vi "DataInit.vi"() -> (3 "output cluster":T1)   [LabVIEW 2011]
uses:
  MainCluster_typdef.ctl
  EC Status Named_typdef.ctl
  EC Statusboolarray2_typdef.ctl
  EC Statusboolarray3_typdef.ctl
  EC Statusboolarray1_typdef.ctl
  EC statusintegerarray_typdef.ctl
  EC statusfloatrarray_typdef.ctl
  LB Status Named_typdef.ctl
  LB Statusboolarray1_typdef.ctl
  LB Statusboolarray2_typdef.ctl
  LB Statusboolarray3_typdef.ctl
  LB statusintegerarray_typdef.ctl
  LB statusfloatrarray_typdef.ctl
  Chamber Selection_typdef.ctl
  GPM Mode_typdef.ctl
panel:
  in  "LB Status Named":T16
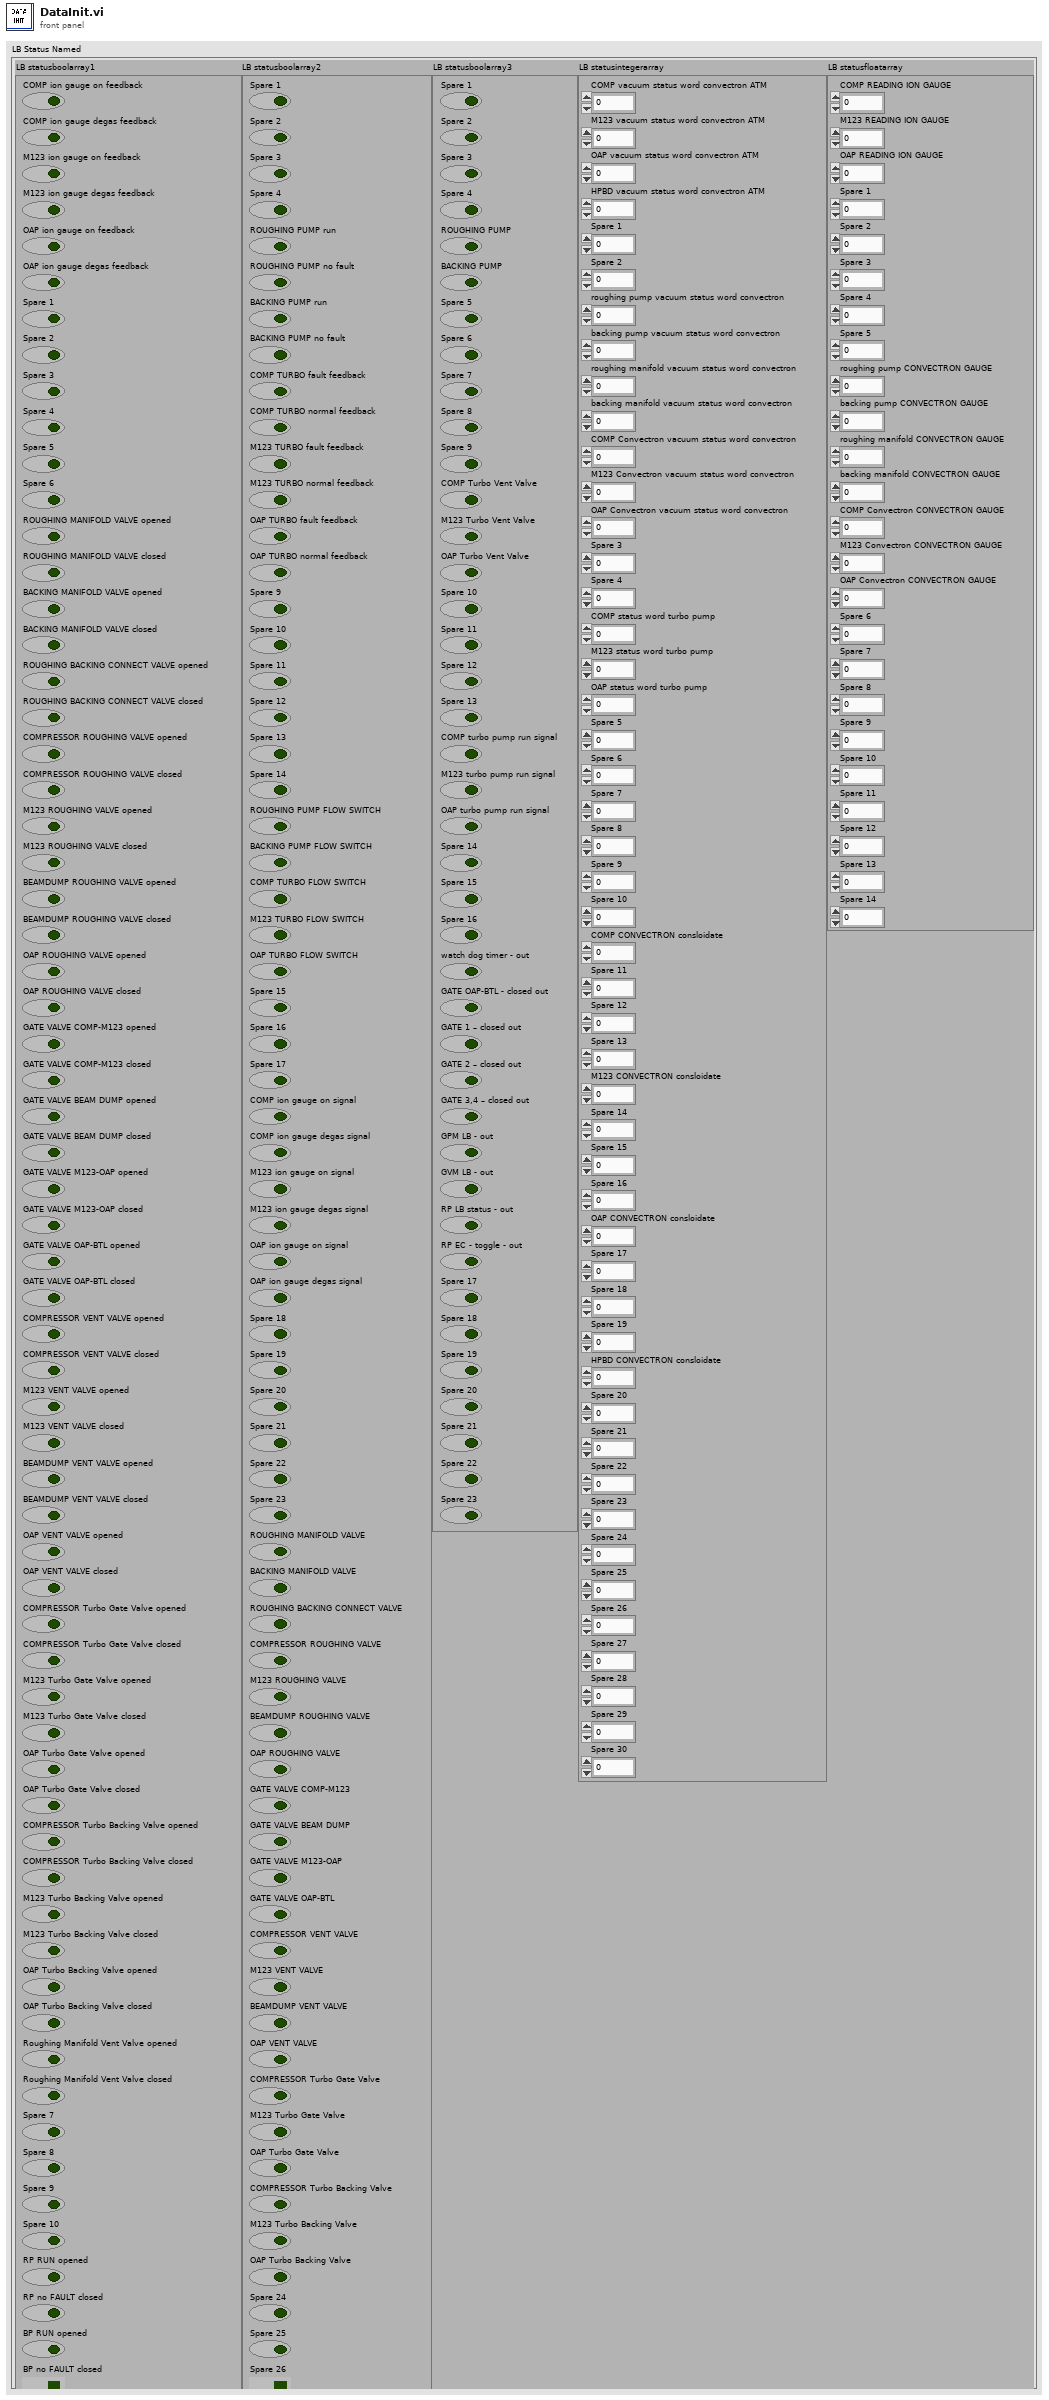
[diagram p1: front panel]
types:
  T1 = typedef "MainCluster_typdef.ctl" = cluster{"Isolate HPBD":bool, "Core":cluster{"Current VI Reference":refnum<vi>, "Close Panel on Exit?":bool}, "Status Display Array":string[], "Connection URLs":cluster{"Source_URL EC":string, "Target_URL EC":string, "Source_URL LB":string, "Target_URL LB":string}, "EC Status":cluster{"bits 2":bool[], "bits 2":bool[], "bits 2":bool[], i32[], "FLOAT NUMBERS 2":sgl[]}, "EC Status Named":T2, "TCPConnection":cluster{"Status TCP Connection EC":refnum<k5>, "Command TCP Connection EC":refnum<k5>, "Status TCP Connection LB":refnum<k5>, "Command TCP Connection LB":refnum<k5>}, "EC Command Cluster":cluster{"boolarray1":cluster{bool, bool, bool, bool, bool, bool, bool, bool, bool, bool, bool, bool, bool, bool, bool, bool}, "boolarray2":cluster{bool, bool, bool, bool, bool, bool, bool, bool, bool, bool, bool, bool, bool, bool, bool, bool}, "boolarray3":cluster{bool, bool, bool, bool, bool, bool, bool, bool, bool, bool, bool, bool, bool, bool, bool, bool}, "boolarray4":cluster{bool, bool, bool, bool, bool, bool, bool, bool, bool, bool, bool, bool, bool, bool, bool, bool}}, "EC Command Named":cluster{"EC Command array 1":cluster{"ROUGHING MANIFOLD VALVE":bool, "BACKING MANIFOLD VALVE":bool, "ROUGHING BACKING CONNECT VALVE":bool, "BTL ROUGHING VALVE":bool, "BTL VENT VALVE":bool, "BTL Turbo Gate Valve":bool, "BTL Turbo Backing Valve":bool, "Roughing Manifold VV":bool, "Backing Manifold VV":bool, "TARGET ROUGHING VALVE":bool, "BTL2 ROUGHING VALVE":bool, "HPD ROUGHING VALVE":bool, "GV BTL-TARGET":bool, "GV TARGET-BTL2":bool, "GV BTL2-HPD":bool, "TARGET VENT VALVE":bool}, " EC Command array 2":cluster{"BTL2 VENT VALVE":bool, "HPD VENT VALVE":bool, "TARGET  Turbo Gate Valve 1":bool, "TARGET  Turbo Gate Valve 2":bool, "BTL2 Turbo Gate Valve":bool, "HPD  Turbo Gate Valve":bool, "TARGET Turbo Backing Valve 1":bool, "TARGET Turbo Backing Valve 2":bool, "BTL2 Turbo Backing Valve":bool, "HPD Turbo Backing Valve":bool, "Spare 1":bool, "Spare 2":bool, "ROUGHING PUMP":bool, "BACKING PUMP":bool, "Spare 3":bool, "Spare 4":bool}, "EC Command array 3":cluster{"Spare 1":bool, "Spare 2":bool, "Spare 3":bool, "BTL Turbo Vent Valve":bool, "TARGET1 Turbo Vent Valve":bool, "TARGET2 Turbo Vent Valve":bool, "BTL2 Turbo Vent Valve":bool, "HPD Turbo Vent Valve":bool, "Spare 4":bool, "Spare 5":bool, "GPM":bool, "GVM":bool, "Spare 6":bool, "BTL turbo pump":bool, "TARGET1 turbo pump":bool, "TARGET2 turbo pump":bool}, "EC Command array 4":cluster{"BLT turbo pump":bool, "HPD turbo pump":bool, "Spare 1":bool, "BTL ION GAUGE ion gauge":bool, "BTL ION GAUGE  ion gauge degas":bool, "TARGET ion gauge":bool, "TARGET ion gauge degas":bool, "BTL2 ion gauge":bool, "BTL2 ion gauge degas":bool, "HPD ion gauge":bool, "HPD ion gauge degas":bool, "Spare 2":bool, "Spare 3":bool, "Spare 4":bool, "Spare 5":bool, "Spare 6":bool}}, "LB Status Named":T8, "LB Status":cluster{"bits 2":bool[], "bits 2":bool[], "bits 2":bool[], i32[], "FLOAT NUMBERS 2":sgl[]}, "LB Command Cluster":cluster{"boolarray1":cluster{bool, bool, bool, bool, bool, bool, bool, bool, bool, bool, bool, bool, bool, bool, bool, bool}, "boolarray2":cluster{bool, bool, bool, bool, bool, bool, bool, bool, bool, bool, bool, bool, bool, bool, bool, bool}, "boolarray3":cluster{bool, bool, bool, bool, bool, bool, bool, bool, bool, bool, bool, bool, bool, bool, bool, bool}, "boolarray4":cluster{bool, bool, bool, bool, bool, bool, bool, bool, bool, bool, bool, bool, bool, bool, bool, bool}}, "LB Command Named":cluster{"LB commandarray1":cluster{"ROUGHING MANIFOLD VALVE":bool, "BACKING MANIFOLD VALVE":bool, "ROUGHING BACKING CONNECT VALVE":bool, "COMPRESSOR ROUGHING VALVE":bool, "M123 ROUGHING VALVE":bool, "BEAMDUMP ROUGHING VALVE":bool, "OAP ROUGHING VALVE":bool, "GATE VALVE COMP-M123":bool, "GATE VALVE BEAM DUMP":bool, "GATE VALVE M123-OAP":bool, "GATE VALVE OAP-BTL":bool, "COMPRESSOR VENT VALVE":bool, "M123 VENT VALVE":bool, "BEAMDUMP VENT VALVE":bool, "OAP VENT VALVE":bool, "COMPRESSOR Turbo Gate Valve":bool}, "LB commandarray2":cluster{"M123 Turbo Gate Valve":bool, "OAP Turbo Gate Valve":bool, "COMPRESSOR Turbo Backing Valve":bool, "M123 Turbo Backing Valve":bool, "OAP Turbo Backing Valve":bool, "Roughing Manifold Vent Valve":bool, "Backing Manifold Vent Valve":bool, "Spare 1":bool, "Spare 2":bool, "Spare 3":bool, "Spare 4":bool, "Spare 5":bool, "ROUGHING PUMP":bool, "BACKING PUMP":bool, "Spare 6":bool, "Spare 7":bool}, "LB commandarray3":cluster{"Spare 1":bool, "Spare 2":bool, "Spare 3":bool, "COMP Turbo Vent Valve":bool, "M123 Turbo Vent Valve":bool, "OAP Turbo Vent Valve":bool, "Spare 4":bool, "Spare 5":bool, "Spare 6":bool, "Spare 7":bool, "GPM":bool, "GVM":bool, "Spare 8":bool, "COMP turbo pump":bool, "M123 turbo pump":bool, "OAP turbo pump":bool}, "LB commandarray4":cluster{"Spare 1":bool, "Spare 2":bool, "Spare 3":bool, "COMP ION GAUGE":bool, "COMP ION GAUGE degas":bool, "M123 ION GAUGE":bool, "M123 ION GAUGE degas":bool, "OAP ION GAUGE":bool, "OAP ION GAUGE degas":bool, "Spare 4":bool, "Spare 5":bool, "Spare 6":bool, "Spare 7":bool, "Spare 8":bool, "Spare 9":bool, "Spare 10":bool}}, "VI Refnum":refnum<vi>, "Chamber Selection":T14, "GPM Mode":T15, "Debug Mode?":bool, "State Sanity Check Array":bool[], "Critical Failures":cluster{"GPM Exit?":bool}, "Comm Ready?":bool, "Status Reconnect Attempt":dbl}
  T2 = typedef "EC Status Named_typdef.ctl" = cluster{"EC statusboolarray2":T3, "EC statusboolarray3":T4, "EC statusboolarray1":T5, "EC statusintegerarray":T6, "EC statusfloatarray":T7}
  T3 = typedef "EC Statusboolarray2_typdef.ctl" = cluster{"Spare 1":bool, "Spare 2":bool, "Spare 3":bool, "Spare 4":bool, "ROUGHING PUMP run opened":bool, "ROUGHING PUMP no fault closed":bool, "BACKING PUMP run opened":bool, "BACKING PUMP no fault closed":bool, "BTL TURBO turbo fault feedback":bool, "BTL TURBO turbo normal feedback":bool, "TARGET 1 TURBO turbo fault feedback":bool, "TARGET 1 TURBO turbo normal feedback":bool, "TARGET 2 TURBO turbo fault feedback":bool, "TARGET 2 TURBO turbo normal feedback":bool, "BTL2 TURBO turbo fault feedback":bool, "BTL2 TURBO turbo normal feedback":bool, "HPD TURBO turbo fault feedback":bool, "HPD TURBO turbo normal feedback":bool, "Spare 5":bool, "Spare 6":bool, "ROUGHING PUMP FLOW SWITCH":bool, "BACKING PUMP FLOW SWITCH":bool, "BTL TURBO FLOW SWITCH":bool, "TARGET 1 TURBO FLOW SWITCH":bool, "TARGET 2 TURBO FLOW SWITCH":bool, "BTL2 TURBO FLOW SWITCH":bool, "HPD TURBO FLOW SWITCH":bool, "Spare 7":bool, "BTL ion gauge on signal":bool, "BTL ion gauge degas signal":bool, "TARGET ion gauge on signal":bool, "TARGET ion gauge degas signal":bool, "BTL2 ion gauge on signal":bool, "BTL2 ion gauge degas signal":bool, "HPD ion gauge on signal":bool, "HPD ion gauge degas signal":bool, "Spare 8":bool, "Spare 9":bool, "Spare 10":bool, "Spare 11":bool, "ROUGHING MANIFOLD VALVE":bool, "BACKING MANIFOLD VALVE":bool, "ROUGHING BACKING CONNECT VALVE":bool, "BTL ROUGHING VALVE":bool, "BTL VENT VALVE":bool, "BTL Turbo Gate Valve":bool, "BTL Turbo Backing Valve":bool, "Roughing Manifold VV":bool, "Backing Manifold VV":bool, "TARGET ROUGHING VALVE":bool, "BTL2 ROUGHING VALVE":bool, "HPD ROUGHING VALVE":bool, "GV BTL-TARGET":bool, "GV TARGET-BTL2":bool, "GV BTL2-HPD":bool, "TARGET VENT VALVE":bool, "BTL2 VENT VALVE":bool, "HPD VENT VALVE":bool, "TARGET  Turbo Gate Valve 1":bool, "TARGET  Turbo Gate Valve 2":bool, "BTL2 Turbo Gate Valve":bool, "HPD  Turbo Gate Valve":bool, "TARGET Turbo Backing Valve 1":bool, "TARGET Turbo Backing Valve 2":bool}
  T4 = typedef "EC Statusboolarray3_typdef.ctl" = cluster{"BTL2 Turbo Backing Valve":bool, "HPD Turbo Backing Valve":bool, "Spare 1":bool, "Spare 2":bool, "Spare 3":bool, "Spare 4":bool, "Spare 5":bool, "Spare 6":bool, "Spare 7":bool, "Spare 8":bool, "Spare 9":bool, "BTL Turbo Vent Valve":bool, "TARGET1 Turbo Vent Valve":bool, "TARGET2 Turbo Vent Valve":bool, "BTL2 Turbo Vent Valve":bool, "HPD Turbo Vent Valve":bool, "Spare 10":bool, "Spare 11":bool, "BTL turbo pump run signal":bool, "TARGET1 turbo pump run signal":bool, "TARGET2 turbo pump run signal":bool, "BTL2 turbo pump run signal":bool, "HPD turbo pump run signal":bool, "Spare 12":bool, "watch dog timer - out":bool, "BTL vented – out":bool, "BTL medvac – out":bool, "BTL hivac – out":bool, "GPM EC - out":bool, "GVM EC - out":bool, "RP EC status - out":bool, "RP LB toggle - out":bool, "GATE ALL - closed out":bool, "Spare 13":bool, "Spare 14":bool, "Spare 15":bool, "Spare 16":bool, "Spare 17":bool, "Spare 18":bool, "Spare 19":bool, "Spare 20":bool, "Spare 21":bool, "Spare 22":bool, "Spare 23":bool, "Spare 24":bool, "Spare 25":bool, "Spare 26":bool, "Spare 27":bool}
  T5 = typedef "EC Statusboolarray1_typdef.ctl" = cluster{"BTL ion gauge on feedback":bool, "BTL ion gauge degas feedback":bool, "TARGET ion gauge on feedback":bool, "TARGET ion gauge degas feedback":bool, "BTL2 ion gauge on feedback":bool, "BTL2 ion gauge degas feedback":bool, "HPD ion gauge on feedback":bool, "HPD ion gauge degas feedback":bool, "Spare 1":bool, "Spare 2":bool, "Spare 3":bool, "Spare 4":bool, "ROUGHING MANIFOLD VALVE opened":bool, "ROUGHING MANIFOLD VALVE closed":bool, "BACKING MANIFOLD VALVE opened":bool, "BACKING MANIFOLD VALVE closed":bool, "ROUGHING BACKING CONNECT VALVE opened":bool, "ROUGHING BACKING CONNECT VALVE closed":bool, "BTL ROUGHING VALVE opened":bool, "BTL ROUGHING VALVE closed":bool, "BTL VENT VALVE opened":bool, "BTL VENT VALVE closed":bool, "BTL Turbo Gate Valve opened":bool, "BTL Turbo Gate Valve closed":bool, "BTL Turbo Backing Valve opened":bool, "BTL Turbo Backing Valve closed":bool, "Roughing Manifold VV opened":bool, "Roughing Manifold VV closed":bool, "Backing Manifold VV opened":bool, "Backing Manifold VV closed":bool, "TARGET ROUGHING VALVE opened":bool, "TARGET ROUGHING VALVE closed":bool, "BTL2 ROUGHING VALVE opened":bool, "BTL2 ROUGHING VALVE closed":bool, "HPD ROUGHING VALVE opened":bool, "HPD ROUGHING VALVE closed":bool, "GV BTL-TARGET opened":bool, "GV BTL-TARGET closed":bool, "GV TARGET-BTL2 opened":bool, "GV TARGET-BTL2 closed":bool, "GV BTL2-HPD opened":bool, "GV BTL2-HPD closed":bool, "TARGET VENT VALVE opened":bool, "TARGET VENT VALVE closed":bool, "BTL2 VENT VALVE opened":bool, "BTL2 VENT VALVE closed":bool, "HPD VENT VALVE opened":bool, "HPD VENT VALVE closed":bool, "TARGET  Turbo Gate Valve 1 opened":bool, "TARGET  Turbo Gate Valve 1 closed":bool, "TARGET  Turbo Gate Valve 2 opened":bool, "TARGET  Turbo Gate Valve 2 closed":bool, "BTL2 Turbo Gate Valve opened":bool, "BTL2 Turbo Gate Valve closed":bool, "HPD  Turbo Gate Valve opened":bool, "HPD  Turbo Gate Valve closed":bool, "TARGET Turbo Backing Valve 1 opened":bool, "TARGET Turbo Backing Valve 1 closed":bool, "TARGET Turbo Backing Valve 2 opened":bool, "TARGET Turbo Backing Valve 2 closed":bool, "BTL2 Turbo Backing Valve opened":bool, "BTL2 Turbo Backing Valve closed":bool, "HPD Turbo Backing Valve opened":bool, "HPD Turbo Backing Valve closed":bool}
  T6 = typedef "EC statusintegerarray_typdef.ctl" = cluster{"BTL vacuum status word convectron ATM":i32, "TARGET vacuum status word convectron ATM 2":i32, "BTL2 vacuum status word convectron ATM 3":i32, "HPD vacuum status word convectron ATM 4":i32, "Spare 1":i32, "Spare 2":i32, "roughing pump vacuum status word convectron":i32, "backing pump vacuum status word convectron":i32, "roughing manifold vacuum status word convectron":i32, "backing manifold vacuum status word convectron":i32, "BTL Convectron vacuum status word convectron":i32, "TARGET1 Convectron vacuum status word convectron":i32, "TARGET2 Convectron vacuum status word convectron":i32, "BTL2 Convectron vacuum status word convectron":i32, "HPD Convectron vacuum status word convectron":i32, "BTL status word turbo pump":i32, "TARGET1 status word turbo pump":i32, "TARGET2 status word turbo pump":i32, "BTL2 status word turbo pump??":i32, "HPD status word turbo pump":i32, "Spare 3":i32, "Spare 4":i32, "Spare 5":i32, "Spare 6":i32, "BTL CONVECTRON Consolidate":i32, "Spare 7":i32, "Spare 8":i32, "Spare 9":i32, "TARGET Consolidate":i32, "Spare 10":i32, "Spare 11":i32, "Spare 12":i32, "BTL2 Consolidate":i32, "Spare 13":i32, "Spare 14":i32, "Spare 15":i32, "HPD Consolidate":i32, "Spare 16":i32, "Spare 17":i32, "Spare 18":i32, "Spare 19":i32, "Spare 20":i32, "Spare 21":i32, "Spare 22":i32, "Spare 23":i32, "Spare 24":i32, "Spare 25":i32, "Spare 26":i32}
  T7 = typedef "EC statusfloatrarray_typdef.ctl" = cluster{"BTL READING ION GAUGE":dbl, "TARGET READING ION GAUGE":dbl, "BTL2 READING ION GAUGE":dbl, "HPD READING ION GAUGE":dbl, "Spare 1":dbl, "Spare 2":dbl, "Spare 3":dbl, "Spare 4":dbl, "roughing pump READING CONVECTRON GAUGE":dbl, "backing pump READING CONVECTRON GAUGE":dbl, "roughing manifold READING CONVECTRON GAUGE":dbl, "backing manifold READING CONVECTRON GAUGE":dbl, "BTL Convectron READING CONVECTRON GAUGE":dbl, "TARGET1 READING CONVECTRON GAUGE":dbl, "TARGET2 READING CONVECTRON GAUGE":dbl, "BTL2 READING CONVECTRON GAUGE":dbl, "HPD READING CONVECTRON GAUGE":dbl, "Spare 5":dbl, "Spare 6":dbl, "Spare 7":dbl, "Spare 8":dbl, "Spare 9":dbl, "Spare 10":dbl, "Spare 11":dbl}
  T8 = typedef "LB Status Named_typdef.ctl" = cluster{"LB statusboolarray1":T9, "LB statusboolarray2":T10, "LB statusboolarray3":T11, "LB statusintegerarray":T12, "LB statusfloatarray":T13}
  T9 = typedef "LB Statusboolarray1_typdef.ctl" = cluster{"COMP ion gauge on feedback":bool, "COMP ion gauge degas feedback":bool, "M123 ion gauge on feedback":bool, "M123 ion gauge degas feedback":bool, "OAP ion gauge on feedback":bool, "OAP ion gauge degas feedback":bool, "Spare 1":bool, "Spare 2":bool, "Spare 3":bool, "Spare 4":bool, "Spare 5":bool, "Spare 6":bool, "ROUGHING MANIFOLD VALVE opened":bool, "ROUGHING MANIFOLD VALVE closed":bool, "BACKING MANIFOLD VALVE opened":bool, "BACKING MANIFOLD VALVE closed":bool, "ROUGHING BACKING CONNECT VALVE opened":bool, "ROUGHING BACKING CONNECT VALVE closed":bool, "COMPRESSOR ROUGHING VALVE opened":bool, "COMPRESSOR ROUGHING VALVE closed":bool, "M123 ROUGHING VALVE opened":bool, "M123 ROUGHING VALVE closed":bool, "BEAMDUMP ROUGHING VALVE opened":bool, "BEAMDUMP ROUGHING VALVE closed":bool, "OAP ROUGHING VALVE opened":bool, "OAP ROUGHING VALVE closed":bool, "GATE VALVE COMP-M123 opened":bool, "GATE VALVE COMP-M123 closed":bool, "GATE VALVE BEAM DUMP opened":bool, "GATE VALVE BEAM DUMP closed":bool, "GATE VALVE M123-OAP opened":bool, "GATE VALVE M123-OAP closed":bool, "GATE VALVE OAP-BTL opened":bool, "GATE VALVE OAP-BTL closed":bool, "COMPRESSOR VENT VALVE opened":bool, "COMPRESSOR VENT VALVE closed":bool, "M123 VENT VALVE opened":bool, "M123 VENT VALVE closed":bool, "BEAMDUMP VENT VALVE opened":bool, "BEAMDUMP VENT VALVE closed":bool, "OAP VENT VALVE opened":bool, "OAP VENT VALVE closed":bool, "COMPRESSOR Turbo Gate Valve opened ":bool, "COMPRESSOR Turbo Gate Valve closed":bool, "M123 Turbo Gate Valve opened":bool, "M123 Turbo Gate Valve closed":bool, "OAP Turbo Gate Valve opened":bool, "OAP Turbo Gate Valve closed":bool, "COMPRESSOR Turbo Backing Valve opened":bool, "COMPRESSOR Turbo Backing Valve closed":bool, "M123 Turbo Backing Valve opened":bool, "M123 Turbo Backing Valve closed":bool, "OAP Turbo Backing Valve opened":bool, "OAP Turbo Backing Valve closed":bool, "Roughing Manifold Vent Valve opened":bool, "Roughing Manifold Vent Valve closed":bool, "Spare 7":bool, "Spare 8":bool, "Spare 9":bool, "Spare 10":bool, "RP RUN opened":bool, "RP no FAULT closed":bool, "BP RUN opened":bool, "BP no FAULT closed":bool}
  T10 = typedef "LB Statusboolarray2_typdef.ctl" = cluster{"Spare 1":bool, "Spare 2":bool, "Spare 3":bool, "Spare 4":bool, "ROUGHING PUMP run":bool, "ROUGHING PUMP no fault":bool, "BACKING PUMP run":bool, "BACKING PUMP no fault":bool, "COMP TURBO fault feedback":bool, "COMP TURBO normal feedback":bool, "M123 TURBO fault feedback":bool, "M123 TURBO normal feedback":bool, "OAP TURBO fault feedback":bool, "OAP TURBO normal feedback":bool, "Spare 9":bool, "Spare 10":bool, "Spare 11":bool, "Spare 12":bool, "Spare 13":bool, "Spare 14":bool, "ROUGHING PUMP FLOW SWITCH":bool, "BACKING PUMP FLOW SWITCH":bool, "COMP TURBO FLOW SWITCH":bool, "M123 TURBO FLOW SWITCH":bool, "OAP TURBO FLOW SWITCH":bool, "Spare 15":bool, "Spare 16":bool, "Spare 17":bool, "COMP ion gauge on signal":bool, "COMP ion gauge degas signal":bool, "M123 ion gauge on signal":bool, "M123 ion gauge degas signal":bool, "OAP ion gauge on signal":bool, "OAP ion gauge degas signal":bool, "Spare 18":bool, "Spare 19":bool, "Spare 20":bool, "Spare 21":bool, "Spare 22":bool, "Spare 23":bool, "ROUGHING MANIFOLD VALVE":bool, "BACKING MANIFOLD VALVE":bool, "ROUGHING BACKING CONNECT VALVE":bool, "COMPRESSOR ROUGHING VALVE":bool, "M123 ROUGHING VALVE":bool, "BEAMDUMP ROUGHING VALVE":bool, "OAP ROUGHING VALVE":bool, "GATE VALVE COMP-M123":bool, "GATE VALVE BEAM DUMP":bool, "GATE VALVE M123-OAP":bool, "GATE VALVE OAP-BTL":bool, "COMPRESSOR VENT VALVE":bool, "M123 VENT VALVE":bool, "BEAMDUMP VENT VALVE":bool, "OAP VENT VALVE":bool, "COMPRESSOR Turbo Gate Valve":bool, "M123 Turbo Gate Valve":bool, "OAP Turbo Gate Valve":bool, "COMPRESSOR Turbo Backing Valve":bool, "M123 Turbo Backing Valve":bool, "OAP Turbo Backing Valve":bool, "Spare 24":bool, "Spare 25":bool, "Spare 26":bool}
  T11 = typedef "LB Statusboolarray3_typdef.ctl" = cluster{"Spare 1":bool, "Spare 2":bool, "Spare 3":bool, "Spare 4":bool, "ROUGHING PUMP":bool, "BACKING PUMP":bool, "Spare 5":bool, "Spare 6":bool, "Spare 7":bool, "Spare 8":bool, "Spare 9":bool, "COMP Turbo Vent Valve":bool, "M123 Turbo Vent Valve":bool, "OAP Turbo Vent Valve":bool, "Spare 10":bool, "Spare 11":bool, "Spare 12":bool, "Spare 13":bool, "COMP turbo pump run signal":bool, "M123 turbo pump run signal":bool, "OAP turbo pump run signal":bool, "Spare 14":bool, "Spare 15":bool, "Spare 16":bool, "watch dog timer - out":bool, "GATE OAP-BTL - closed out":bool, "GATE 1 – closed out":bool, "GATE 2 – closed out":bool, "GATE 3,4 – closed out":bool, "GPM LB - out":bool, "GVM LB - out":bool, "RP LB status - out":bool, "RP EC - toggle - out":bool, "Spare 17":bool, "Spare 18":bool, "Spare 19":bool, "Spare 20":bool, "Spare 21":bool, "Spare 22":bool, "Spare 23":bool}
  T12 = typedef "LB statusintegerarray_typdef.ctl" = cluster{"COMP vacuum status word convectron ATM":i32, "M123 vacuum status word convectron ATM":i32, "OAP vacuum status word convectron ATM":i32, "HPBD vacuum status word convectron ATM":i32, "Spare 1":i32, "Spare 2":i32, "roughing pump vacuum status word convectron":i32, "backing pump vacuum status word convectron":i32, "roughing manifold vacuum status word convectron":i32, "backing manifold vacuum status word convectron":i32, "COMP Convectron vacuum status word convectron":i32, "M123 Convectron vacuum status word convectron":i32, "OAP Convectron vacuum status word convectron":i32, "Spare 3":i32, "Spare 4":i32, "COMP status word turbo pump":i32, "M123 status word turbo pump":i32, "OAP status word turbo pump":i32, "Spare 5":i32, "Spare 6":i32, "Spare 7":i32, "Spare 8":i32, "Spare 9":i32, "Spare 10":i32, "COMP CONVECTRON consloidate":i32, "Spare 11":i32, "Spare 12":i32, "Spare 13":i32, "M123 CONVECTRON consloidate":i32, "Spare 14":i32, "Spare 15":i32, "Spare 16":i32, "OAP CONVECTRON consloidate":i32, "Spare 17":i32, "Spare 18":i32, "Spare 19":i32, "HPBD CONVECTRON consloidate":i32, "Spare 20":i32, "Spare 21":i32, "Spare 22":i32, "Spare 23":i32, "Spare 24":i32, "Spare 25":i32, "Spare 26":i32, "Spare 27":i32, "Spare 28":i32, "Spare 29":i32, "Spare 30":i32}
  T13 = typedef "LB statusfloatrarray_typdef.ctl" = cluster{"COMP READING ION GAUGE":dbl, "M123 READING ION GAUGE":dbl, "OAP READING ION GAUGE":dbl, "Spare 1":i32, "Spare 2":i32, "Spare 3":i32, "Spare 4":i32, "Spare 5":i32, "roughing pump CONVECTRON GAUGE":dbl, "backing pump CONVECTRON GAUGE":dbl, "roughing manifold CONVECTRON GAUGE":dbl, "backing manifold CONVECTRON GAUGE":dbl, "COMP Convectron CONVECTRON GAUGE":dbl, "M123 Convectron CONVECTRON GAUGE":dbl, "OAP Convectron CONVECTRON GAUGE":dbl, "Spare 6":i32, "Spare 7":i32, "Spare 8":i32, "Spare 9":i32, "Spare 10":i32, "Spare 11":i32, "Spare 12":i32, "Spare 13":i32, "Spare 14":i32}
  T14 = typedef "Chamber Selection_typdef.ctl" = cluster{"COMP":bool, "M123":bool, "HPBD":bool, "OAP":bool, "BTL":bool, "TARGET":bool, "BTL2":bool, "HPD":bool}
  T15 = typedef "GPM Mode_typdef.ctl" = enum16{"Complete Global Pump Mode", "Selected Global Pump Mode"}
  T16 = cluster{"LB statusboolarray1":cluster{"COMP ion gauge on feedback":bool, "COMP ion gauge degas feedback":bool, "M123 ion gauge on feedback":bool, "M123 ion gauge degas feedback":bool, "OAP ion gauge on feedback":bool, "OAP ion gauge degas feedback":bool, "Spare 1":bool, "Spare 2":bool, "Spare 3":bool, "Spare 4":bool, "Spare 5":bool, "Spare 6":bool, "ROUGHING MANIFOLD VALVE opened":bool, "ROUGHING MANIFOLD VALVE closed":bool, "BACKING MANIFOLD VALVE opened":bool, "BACKING MANIFOLD VALVE closed":bool, "ROUGHING BACKING CONNECT VALVE opened":bool, "ROUGHING BACKING CONNECT VALVE closed":bool, "COMPRESSOR ROUGHING VALVE opened":bool, "COMPRESSOR ROUGHING VALVE closed":bool, "M123 ROUGHING VALVE opened":bool, "M123 ROUGHING VALVE closed":bool, "BEAMDUMP ROUGHING VALVE opened":bool, "BEAMDUMP ROUGHING VALVE closed":bool, "OAP ROUGHING VALVE opened":bool, "OAP ROUGHING VALVE closed":bool, "GATE VALVE COMP-M123 opened":bool, "GATE VALVE COMP-M123 closed":bool, "GATE VALVE BEAM DUMP opened":bool, "GATE VALVE BEAM DUMP closed":bool, "GATE VALVE M123-OAP opened":bool, "GATE VALVE M123-OAP closed":bool, "GATE VALVE OAP-BTL opened":bool, "GATE VALVE OAP-BTL closed":bool, "COMPRESSOR VENT VALVE opened":bool, "COMPRESSOR VENT VALVE closed":bool, "M123 VENT VALVE opened":bool, "M123 VENT VALVE closed":bool, "BEAMDUMP VENT VALVE opened":bool, "BEAMDUMP VENT VALVE closed":bool, "OAP VENT VALVE opened":bool, "OAP VENT VALVE closed":bool, "COMPRESSOR Turbo Gate Valve opened ":bool, "COMPRESSOR Turbo Gate Valve closed":bool, "M123 Turbo Gate Valve opened":bool, "M123 Turbo Gate Valve closed":bool, "OAP Turbo Gate Valve opened":bool, "OAP Turbo Gate Valve closed":bool, "COMPRESSOR Turbo Backing Valve opened":bool, "COMPRESSOR Turbo Backing Valve closed":bool, "M123 Turbo Backing Valve opened":bool, "M123 Turbo Backing Valve closed":bool, "OAP Turbo Backing Valve opened":bool, "OAP Turbo Backing Valve closed":bool, "Roughing Manifold Vent Valve opened":bool, "Roughing Manifold Vent Valve closed":bool, "Spare 7":bool, "Spare 8":bool, "Spare 9":bool, "Spare 10":bool, "RP RUN opened":bool, "RP no FAULT closed":bool, "BP RUN opened":bool, "BP no FAULT closed":bool}, "LB statusboolarray2":cluster{"Spare 1":bool, "Spare 2":bool, "Spare 3":bool, "Spare 4":bool, "ROUGHING PUMP run":bool, "ROUGHING PUMP no fault":bool, "BACKING PUMP run":bool, "BACKING PUMP no fault":bool, "COMP TURBO fault feedback":bool, "COMP TURBO normal feedback":bool, "M123 TURBO fault feedback":bool, "M123 TURBO normal feedback":bool, "OAP TURBO fault feedback":bool, "OAP TURBO normal feedback":bool, "Spare 9":bool, "Spare 10":bool, "Spare 11":bool, "Spare 12":bool, "Spare 13":bool, "Spare 14":bool, "ROUGHING PUMP FLOW SWITCH":bool, "BACKING PUMP FLOW SWITCH":bool, "COMP TURBO FLOW SWITCH":bool, "M123 TURBO FLOW SWITCH":bool, "OAP TURBO FLOW SWITCH":bool, "Spare 15":bool, "Spare 16":bool, "Spare 17":bool, "COMP ion gauge on signal":bool, "COMP ion gauge degas signal":bool, "M123 ion gauge on signal":bool, "M123 ion gauge degas signal":bool, "OAP ion gauge on signal":bool, "OAP ion gauge degas signal":bool, "Spare 18":bool, "Spare 19":bool, "Spare 20":bool, "Spare 21":bool, "Spare 22":bool, "Spare 23":bool, "ROUGHING MANIFOLD VALVE":bool, "BACKING MANIFOLD VALVE":bool, "ROUGHING BACKING CONNECT VALVE":bool, "COMPRESSOR ROUGHING VALVE":bool, "M123 ROUGHING VALVE":bool, "BEAMDUMP ROUGHING VALVE":bool, "OAP ROUGHING VALVE":bool, "GATE VALVE COMP-M123":bool, "GATE VALVE BEAM DUMP":bool, "GATE VALVE M123-OAP":bool, "GATE VALVE OAP-BTL":bool, "COMPRESSOR VENT VALVE":bool, "M123 VENT VALVE":bool, "BEAMDUMP VENT VALVE":bool, "OAP VENT VALVE":bool, "COMPRESSOR Turbo Gate Valve":bool, "M123 Turbo Gate Valve":bool, "OAP Turbo Gate Valve":bool, "COMPRESSOR Turbo Backing Valve":bool, "M123 Turbo Backing Valve":bool, "OAP Turbo Backing Valve":bool, "Spare 24":bool, "Spare 25":bool, "Spare 26":bool}, "LB statusboolarray3":cluster{"Spare 1":bool, "Spare 2":bool, "Spare 3":bool, "Spare 4":bool, "ROUGHING PUMP":bool, "BACKING PUMP":bool, "Spare 5":bool, "Spare 6":bool, "Spare 7":bool, "Spare 8":bool, "Spare 9":bool, "COMP Turbo Vent Valve":bool, "M123 Turbo Vent Valve":bool, "OAP Turbo Vent Valve":bool, "Spare 10":bool, "Spare 11":bool, "Spare 12":bool, "Spare 13":bool, "COMP turbo pump run signal":bool, "M123 turbo pump run signal":bool, "OAP turbo pump run signal":bool, "Spare 14":bool, "Spare 15":bool, "Spare 16":bool, "watch dog timer - out":bool, "GATE OAP-BTL - closed out":bool, "GATE 1 – closed out":bool, "GATE 2 – closed out":bool, "GATE 3,4 – closed out":bool, "GPM LB - out":bool, "GVM LB - out":bool, "RP LB status - out":bool, "RP EC - toggle - out":bool, "Spare 17":bool, "Spare 18":bool, "Spare 19":bool, "Spare 20":bool, "Spare 21":bool, "Spare 22":bool, "Spare 23":bool}, "LB statusintegerarray":cluster{"COMP vacuum status word convectron ATM":i32, "M123 vacuum status word convectron ATM":i32, "OAP vacuum status word convectron ATM":i32, "HPBD vacuum status word convectron ATM":i32, "Spare 1":i32, "Spare 2":i32, "roughing pump vacuum status word convectron":i32, "backing pump vacuum status word convectron":i32, "roughing manifold vacuum status word convectron":i32, "backing manifold vacuum status word convectron":i32, "COMP Convectron vacuum status word convectron":i32, "M123 Convectron vacuum status word convectron":i32, "OAP Convectron vacuum status word convectron":i32, "Spare 3":i32, "Spare 4":i32, "COMP status word turbo pump":i32, "M123 status word turbo pump":i32, "OAP status word turbo pump":i32, "Spare 5":i32, "Spare 6":i32, "Spare 7":i32, "Spare 8":i32, "Spare 9":i32, "Spare 10":i32, "COMP CONVECTRON consloidate":i32, "Spare 11":i32, "Spare 12":i32, "Spare 13":i32, "M123 CONVECTRON consloidate":i32, "Spare 14":i32, "Spare 15":i32, "Spare 16":i32, "OAP CONVECTRON consloidate":i32, "Spare 17":i32, "Spare 18":i32, "Spare 19":i32, "HPBD CONVECTRON consloidate":i32, "Spare 20":i32, "Spare 21":i32, "Spare 22":i32, "Spare 23":i32, "Spare 24":i32, "Spare 25":i32, "Spare 26":i32, "Spare 27":i32, "Spare 28":i32, "Spare 29":i32, "Spare 30":i32}, "LB statusfloatarray":cluster{"COMP READING ION GAUGE":dbl, "M123 READING ION GAUGE":dbl, "OAP READING ION GAUGE":dbl, "Spare 1":i32, "Spare 2":i32, "Spare 3":i32, "Spare 4":i32, "Spare 5":i32, "roughing pump CONVECTRON GAUGE":dbl, "backing pump CONVECTRON GAUGE":dbl, "roughing manifold CONVECTRON GAUGE":dbl, "backing manifold CONVECTRON GAUGE":dbl, "COMP Convectron CONVECTRON GAUGE":dbl, "M123 Convectron CONVECTRON GAUGE":dbl, "OAP Convectron CONVECTRON GAUGE":dbl, "Spare 6":i32, "Spare 7":i32, "Spare 8":i32, "Spare 9":i32, "Spare 10":i32, "Spare 11":i32, "Spare 12":i32, "Spare 13":i32, "Spare 14":i32}}
  T17 = cluster{"LB commandarray1":cluster{"ROUGHING MANIFOLD VALVE":bool, "BACKING MANIFOLD VALVE":bool, "ROUGHING BACKING CONNECT VALVE":bool, "COMPRESSOR ROUGHING VALVE":bool, "M123 ROUGHING VALVE":bool, "BEAMDUMP ROUGHING VALVE":bool, "OAP ROUGHING VALVE":bool, "GATE VALVE COMP-M123":bool, "GATE VALVE BEAM DUMP":bool, "GATE VALVE M123-OAP":bool, "GATE VALVE OAP-BTL":bool, "COMPRESSOR VENT VALVE":bool, "M123 VENT VALVE":bool, "BEAMDUMP VENT VALVE":bool, "OAP VENT VALVE":bool, "COMPRESSOR Turbo Gate Valve":bool}, "LB commandarray2":cluster{"M123 Turbo Gate Valve":bool, "OAP Turbo Gate Valve":bool, "COMPRESSOR Turbo Backing Valve":bool, "M123 Turbo Backing Valve":bool, "OAP Turbo Backing Valve":bool, "Roughing Manifold Vent Valve":bool, "Backing Manifold Vent Valve":bool, "Spare 1":bool, "Spare 2":bool, "Spare 3":bool, "Spare 4":bool, "Spare 5":bool, "ROUGHING PUMP":bool, "BACKING PUMP":bool, "Spare 6":bool, "Spare 7":bool}, "LB commandarray3":cluster{"Spare 1":bool, "Spare 2":bool, "Spare 3":bool, "COMP Turbo Vent Valve":bool, "M123 Turbo Vent Valve":bool, "OAP Turbo Vent Valve":bool, "Spare 4":bool, "Spare 5":bool, "Spare 6":bool, "Spare 7":bool, "GPM":bool, "GVM":bool, "Spare 8":bool, "COMP turbo pump":bool, "M123 turbo pump":bool, "OAP turbo pump":bool}, "LB commandarray4":cluster{"Spare 1":bool, "Spare 2":bool, "Spare 3":bool, "COMP ION GAUGE":bool, "COMP ION GAUGE degas":bool, "M123 ION GAUGE":bool, "M123 ION GAUGE degas":bool, "OAP ION GAUGE":bool, "OAP ION GAUGE degas":bool, "Spare 4":bool, "Spare 5":bool, "Spare 6":bool, "Spare 7":bool, "Spare 8":bool, "Spare 9":bool, "Spare 10":bool}}
  T18 = cluster{"EC statusboolarray2":cluster{"Spare 1":bool, "Spare 2":bool, "Spare 3":bool, "Spare 4":bool, "ROUGHING PUMP run opened":bool, "ROUGHING PUMP no fault closed":bool, "BACKING PUMP run opened":bool, "BACKING PUMP no fault closed":bool, "BTL TURBO turbo fault feedback":bool, "BTL TURBO turbo normal feedback":bool, "TARGET 1 TURBO turbo fault feedback":bool, "TARGET 1 TURBO turbo normal feedback":bool, "TARGET 2 TURBO turbo fault feedback":bool, "TARGET 2 TURBO turbo normal feedback":bool, "BTL2 TURBO turbo fault feedback":bool, "BTL2 TURBO turbo normal feedback":bool, "HPD TURBO turbo fault feedback":bool, "HPD TURBO turbo normal feedback":bool, "Spare 5":bool, "Spare 6":bool, "ROUGHING PUMP FLOW SWITCH":bool, "BACKING PUMP FLOW SWITCH":bool, "BTL TURBO FLOW SWITCH":bool, "TARGET 1 TURBO FLOW SWITCH":bool, "TARGET 2 TURBO FLOW SWITCH":bool, "BTL2 TURBO FLOW SWITCH":bool, "HPD TURBO FLOW SWITCH":bool, "Spare 7":bool, "BTL ion gauge on signal":bool, "BTL ion gauge degas signal":bool, "TARGET ion gauge on signal":bool, "TARGET ion gauge degas signal":bool, "BTL2 ion gauge on signal":bool, "BTL2 ion gauge degas signal":bool, "HPD ion gauge on signal":bool, "HPD ion gauge degas signal":bool, "Spare 8":bool, "Spare 9":bool, "Spare 10":bool, "Spare 11":bool, "ROUGHING MANIFOLD VALVE":bool, "BACKING MANIFOLD VALVE":bool, "ROUGHING BACKING CONNECT VALVE":bool, "BTL ROUGHING VALVE":bool, "BTL VENT VALVE":bool, "BTL Turbo Gate Valve":bool, "BTL Turbo Backing Valve":bool, "Roughing Manifold VV":bool, "Backing Manifold VV":bool, "TARGET ROUGHING VALVE":bool, "BTL2 ROUGHING VALVE":bool, "HPD ROUGHING VALVE":bool, "GV BTL-TARGET":bool, "GV TARGET-BTL2":bool, "GV BTL2-HPD":bool, "TARGET VENT VALVE":bool, "BTL2 VENT VALVE":bool, "HPD VENT VALVE":bool, "TARGET  Turbo Gate Valve 1":bool, "TARGET  Turbo Gate Valve 2":bool, "BTL2 Turbo Gate Valve":bool, "HPD  Turbo Gate Valve":bool, "TARGET Turbo Backing Valve 1":bool, "TARGET Turbo Backing Valve 2":bool}, "EC statusboolarray3":cluster{"BTL2 Turbo Backing Valve":bool, "HPD Turbo Backing Valve":bool, "Spare 1":bool, "Spare 2":bool, "Spare 3":bool, "Spare 4":bool, "Spare 5":bool, "Spare 6":bool, "Spare 7":bool, "Spare 8":bool, "Spare 9":bool, "BTL Turbo Vent Valve":bool, "TARGET1 Turbo Vent Valve":bool, "TARGET2 Turbo Vent Valve":bool, "BTL2 Turbo Vent Valve":bool, "HPD Turbo Vent Valve":bool, "Spare 10":bool, "Spare 11":bool, "BTL turbo pump run signal":bool, "TARGET1 turbo pump run signal":bool, "TARGET2 turbo pump run signal":bool, "BTL2 turbo pump run signal":bool, "HPD turbo pump run signal":bool, "Spare 12":bool, "watch dog timer - out":bool, "BTL vented – out":bool, "BTL medvac – out":bool, "BTL hivac – out":bool, "GPM EC - out":bool, "GVM EC - out":bool, "RP EC status - out":bool, "RP LB toggle - out":bool, "GATE ALL - closed out":bool, "Spare 13":bool, "Spare 14":bool, "Spare 15":bool, "Spare 16":bool, "Spare 17":bool, "Spare 18":bool, "Spare 19":bool, "Spare 20":bool, "Spare 21":bool, "Spare 22":bool, "Spare 23":bool, "Spare 24":bool, "Spare 25":bool, "Spare 26":bool, "Spare 27":bool}, "EC statusboolarray1":cluster{"BTL ion gauge on feedback":bool, "BTL ion gauge degas feedback":bool, "TARGET ion gauge on feedback":bool, "TARGET ion gauge degas feedback":bool, "BTL2 ion gauge on feedback":bool, "BTL2 ion gauge degas feedback":bool, "HPD ion gauge on feedback":bool, "HPD ion gauge degas feedback":bool, "Spare 1":bool, "Spare 2":bool, "Spare 3":bool, "Spare 4":bool, "ROUGHING MANIFOLD VALVE opened":bool, "ROUGHING MANIFOLD VALVE closed":bool, "BACKING MANIFOLD VALVE opened":bool, "BACKING MANIFOLD VALVE closed":bool, "ROUGHING BACKING CONNECT VALVE opened":bool, "ROUGHING BACKING CONNECT VALVE closed":bool, "BTL ROUGHING VALVE opened":bool, "BTL ROUGHING VALVE closed":bool, "BTL VENT VALVE opened":bool, "BTL VENT VALVE closed":bool, "BTL Turbo Gate Valve opened":bool, "BTL Turbo Gate Valve closed":bool, "BTL Turbo Backing Valve opened":bool, "BTL Turbo Backing Valve closed":bool, "Roughing Manifold VV opened":bool, "Roughing Manifold VV closed":bool, "Backing Manifold VV opened":bool, "Backing Manifold VV closed":bool, "TARGET ROUGHING VALVE opened":bool, "TARGET ROUGHING VALVE closed":bool, "BTL2 ROUGHING VALVE opened":bool, "BTL2 ROUGHING VALVE closed":bool, "HPD ROUGHING VALVE opened":bool, "HPD ROUGHING VALVE closed":bool, "GV BTL-TARGET opened":bool, "GV BTL-TARGET closed":bool, "GV TARGET-BTL2 opened":bool, "GV TARGET-BTL2 closed":bool, "GV BTL2-HPD opened":bool, "GV BTL2-HPD closed":bool, "TARGET VENT VALVE opened":bool, "TARGET VENT VALVE closed":bool, "BTL2 VENT VALVE opened":bool, "BTL2 VENT VALVE closed":bool, "HPD VENT VALVE opened":bool, "HPD VENT VALVE closed":bool, "TARGET  Turbo Gate Valve 1 opened":bool, "TARGET  Turbo Gate Valve 1 closed":bool, "TARGET  Turbo Gate Valve 2 opened":bool, "TARGET  Turbo Gate Valve 2 closed":bool, "BTL2 Turbo Gate Valve opened":bool, "BTL2 Turbo Gate Valve closed":bool, "HPD  Turbo Gate Valve opened":bool, "HPD  Turbo Gate Valve closed":bool, "TARGET Turbo Backing Valve 1 opened":bool, "TARGET Turbo Backing Valve 1 closed":bool, "TARGET Turbo Backing Valve 2 opened":bool, "TARGET Turbo Backing Valve 2 closed":bool, "BTL2 Turbo Backing Valve opened":bool, "BTL2 Turbo Backing Valve closed":bool, "HPD Turbo Backing Valve opened":bool, "HPD Turbo Backing Valve closed":bool}, "EC statusintegerarray":cluster{"BTL vacuum status word convectron ATM":i32, "TARGET vacuum status word convectron ATM 2":i32, "BTL2 vacuum status word convectron ATM 3":i32, "HPD vacuum status word convectron ATM 4":i32, "Spare 1":i32, "Spare 2":i32, "roughing pump vacuum status word convectron":i32, "backing pump vacuum status word convectron":i32, "roughing manifold vacuum status word convectron":i32, "backing manifold vacuum status word convectron":i32, "BTL Convectron vacuum status word convectron":i32, "TARGET1 Convectron vacuum status word convectron":i32, "TARGET2 Convectron vacuum status word convectron":i32, "BTL2 Convectron vacuum status word convectron":i32, "HPD Convectron vacuum status word convectron":i32, "BTL status word turbo pump":i32, "TARGET1 status word turbo pump":i32, "TARGET2 status word turbo pump":i32, "BTL2 status word turbo pump??":i32, "HPD status word turbo pump":i32, "Spare 3":i32, "Spare 4":i32, "Spare 5":i32, "Spare 6":i32, "BTL CONVECTRON Consolidate":i32, "Spare 7":i32, "Spare 8":i32, "Spare 9":i32, "TARGET Consolidate":i32, "Spare 10":i32, "Spare 11":i32, "Spare 12":i32, "BTL2 Consolidate":i32, "Spare 13":i32, "Spare 14":i32, "Spare 15":i32, "HPD Consolidate":i32, "Spare 16":i32, "Spare 17":i32, "Spare 18":i32, "Spare 19":i32, "Spare 20":i32, "Spare 21":i32, "Spare 22":i32, "Spare 23":i32, "Spare 24":i32, "Spare 25":i32, "Spare 26":i32}, "EC statusfloatarray":cluster{"BTL READING ION GAUGE":dbl, "TARGET READING ION GAUGE":dbl, "BTL2 READING ION GAUGE":dbl, "HPD READING ION GAUGE":dbl, "Spare 1":dbl, "Spare 2":dbl, "Spare 3":dbl, "Spare 4":dbl, "roughing pump READING CONVECTRON GAUGE":dbl, "backing pump READING CONVECTRON GAUGE":dbl, "roughing manifold READING CONVECTRON GAUGE":dbl, "backing manifold READING CONVECTRON GAUGE":dbl, "BTL Convectron READING CONVECTRON GAUGE":dbl, "TARGET1 READING CONVECTRON GAUGE":dbl, "TARGET2 READING CONVECTRON GAUGE":dbl, "BTL2 READING CONVECTRON GAUGE":dbl, "HPD READING CONVECTRON GAUGE":dbl, "Spare 5":dbl, "Spare 6":dbl, "Spare 7":dbl, "Spare 8":dbl, "Spare 9":dbl, "Spare 10":dbl, "Spare 11":dbl}}
  T19 = cluster{"EC Command array 1":cluster{"ROUGHING MANIFOLD VALVE":bool, "BACKING MANIFOLD VALVE":bool, "ROUGHING BACKING CONNECT VALVE":bool, "BTL ROUGHING VALVE":bool, "BTL VENT VALVE":bool, "BTL Turbo Gate Valve":bool, "BTL Turbo Backing Valve":bool, "Roughing Manifold VV":bool, "Backing Manifold VV":bool, "TARGET ROUGHING VALVE":bool, "BTL2 ROUGHING VALVE":bool, "HPD ROUGHING VALVE":bool, "GV BTL-TARGET":bool, "GV TARGET-BTL2":bool, "GV BTL2-HPD":bool, "TARGET VENT VALVE":bool}, " EC Command array 2":cluster{"BTL2 VENT VALVE":bool, "HPD VENT VALVE":bool, "TARGET  Turbo Gate Valve 1":bool, "TARGET  Turbo Gate Valve 2":bool, "BTL2 Turbo Gate Valve":bool, "HPD  Turbo Gate Valve":bool, "TARGET Turbo Backing Valve 1":bool, "TARGET Turbo Backing Valve 2":bool, "BTL2 Turbo Backing Valve":bool, "HPD Turbo Backing Valve":bool, "Spare 1":bool, "Spare 2":bool, "ROUGHING PUMP":bool, "BACKING PUMP":bool, "Spare 3":bool, "Spare 4":bool}, "EC Command array 3":cluster{"Spare 1":bool, "Spare 2":bool, "Spare 3":bool, "BTL Turbo Vent Valve":bool, "TARGET1 Turbo Vent Valve":bool, "TARGET2 Turbo Vent Valve":bool, "BTL2 Turbo Vent Valve":bool, "HPD Turbo Vent Valve":bool, "Spare 4":bool, "Spare 5":bool, "GPM":bool, "GVM":bool, "Spare 6":bool, "BTL turbo pump":bool, "TARGET1 turbo pump":bool, "TARGET2 turbo pump":bool}, "EC Command array 4":cluster{"BLT turbo pump":bool, "HPD turbo pump":bool, "Spare 1":bool, "BTL ION GAUGE ion gauge":bool, "BTL ION GAUGE  ion gauge degas":bool, "TARGET ion gauge":bool, "TARGET ion gauge degas":bool, "BTL2 ion gauge":bool, "BTL2 ion gauge degas":bool, "HPD ion gauge":bool, "HPD ion gauge degas":bool, "Spare 2":bool, "Spare 3":bool, "Spare 4":bool, "Spare 5":bool, "Spare 6":bool}}
  T20 = cluster{"boolarray1":cluster{bool, bool, bool, bool, bool, bool, bool, bool, bool, bool, bool, bool, bool, bool, bool, bool}, "boolarray2":cluster{bool, bool, bool, bool, bool, bool, bool, bool, bool, bool, bool, bool, bool, bool, bool, bool}, "boolarray3":cluster{bool, bool, bool, bool, bool, bool, bool, bool, bool, bool, bool, bool, bool, bool, bool, bool}, "boolarray4":cluster{bool, bool, bool, bool, bool, bool, bool, bool, bool, bool, bool, bool, bool, bool, bool, bool}}
  T21 = cluster{"bits 2":bool[], "bits 2":bool[], "bits 2":bool[], i32[], "FLOAT NUMBERS 2":sgl[]}
  T22 = cluster{"Source_URL EC":string, "Target_URL EC":string, "Source_URL LB":string, "Target_URL LB":string}
  T23 = cluster{"Status TCP Connection EC":refnum<k5>, "Command TCP Connection EC":refnum<k5>, "Status TCP Connection LB":refnum<k5>, "Command TCP Connection LB":refnum<k5>}
  T24 = cluster{"Current VI Reference":refnum<vi>, "Close Panel on Exit?":bool}
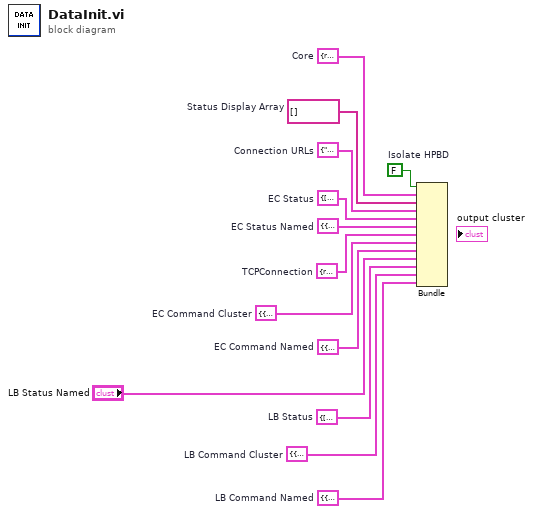
[diagram p0: block diagram]
diagram:
  w1 = FALSE  # Isolate HPBD
  w2 = string[] []  # Status Display Array
  w3 = T17 {"LB commandarray1"={"ROUGHING MANIFOLD VALVE"=FALSE, "BACKING MANIFOLD VALVE"=FALSE, "ROUGHING BACKING CONNECT VALVE"=FALSE, "COMPRESSOR ROUGHING VALVE"=FALSE, "M123 ROUGHING VALVE"=FALSE, "BEAMDUMP ROUGHING VALVE"=FALSE, "OAP ROUGHING VALVE"=FALSE, "GATE VALVE COMP-M123"=FALSE, "GATE VALVE BEAM DUMP"=FALSE, "GATE VALVE M123-OAP"=FALSE, "GATE VALVE OAP-BTL"=FALSE, "COMPRESSOR VENT VALVE"=FALSE, "M123 VENT VALVE"=FALSE, "BEAMDUMP VENT VALVE"=FALSE, "OAP VENT VALVE"=FALSE, "COMPRESSOR Turbo Gate Valve"=FALSE}, "LB commandarray2"={"M123 Turbo Gate Valve"=FALSE, "OAP Turbo Gate Valve"=FALSE, "COMPRESSOR Turbo Backing Valve"=FALSE, "M123 Turbo Backing Valve"=FALSE, "OAP Turbo Backing Valve"=FALSE, "Roughing Manifold Vent Valve"=FALSE, "Backing Manifold Vent Valve"=FALSE, "Spare 1"=FALSE, "Spare 2"=FALSE, "Spare 3"=FALSE, "Spare 4"=FALSE, "Spare 5"=FALSE, "ROUGHING PUMP"=FALSE, "BACKING PUMP"=FALSE, "Spare 6"=FALSE, "Spare 7"=FALSE}, "LB commandarray3"={"Spare 1"=FALSE, "Spare 2"=FALSE, "Spare 3"=FALSE, "COMP Turbo Vent Valve"=FALSE, "M123 Turbo Vent Valve"=FALSE, "OAP Turbo Vent Valve"=FALSE, "Spare 4"=FALSE, "Spare 5"=FALSE, "Spare 6"=FALSE, "Spare 7"=FALSE, "GPM"=FALSE, "GVM"=FALSE, "Spare 8"=FALSE, "COMP turbo pump"=FALSE, "M123 turbo pump"=FALSE, "OAP turbo pump"=FALSE}, "LB commandarray4"={"Spare 1"=FALSE, "Spare 2"=FALSE, "Spare 3"=FALSE, "COMP ION GAUGE"=FALSE, "COMP ION GAUGE degas"=FALSE, "M123 ION GAUGE"=FALSE, "M123 ION GAUGE degas"=FALSE, "OAP ION GAUGE"=FALSE, "OAP ION GAUGE degas"=FALSE, "Spare 4"=FALSE, "Spare 5"=FALSE, "Spare 6"=FALSE, "Spare 7"=FALSE, "Spare 8"=FALSE, "Spare 9"=FALSE, "Spare 10"=FALSE}}  # LB Command Named
  w9 = T18 {"EC statusboolarray2"={"Spare 1"=FALSE, "Spare 2"=FALSE, "Spare 3"=FALSE, "Spare 4"=FALSE, "ROUGHING PUMP run opened"=FALSE, "ROUGHING PUMP no fault closed"=FALSE, "BACKING PUMP run opened"=FALSE, "BACKING PUMP no fault closed"=FALSE, "BTL TURBO turbo fault feedback"=FALSE, "BTL TURBO turbo normal feedback"=FALSE, "TARGET 1 TURBO turbo fault feedback"=FALSE, "TARGET 1 TURBO turbo normal feedback"=FALSE, "TARGET 2 TURBO turbo fault feedback"=FALSE, "TARGET 2 TURBO turbo normal feedback"=FALSE, "BTL2 TURBO turbo fault feedback"=FALSE, "BTL2 TURBO turbo normal feedback"=FALSE, "HPD TURBO turbo fault feedback"=FALSE, "HPD TURBO turbo normal feedback"=FALSE, "Spare 5"=FALSE, "Spare 6"=FALSE, "ROUGHING PUMP FLOW SWITCH"=FALSE, "BACKING PUMP FLOW SWITCH"=FALSE, "BTL TURBO FLOW SWITCH"=FALSE, "TARGET 1 TURBO FLOW SWITCH"=FALSE, "TARGET 2 TURBO FLOW SWITCH"=FALSE, "BTL2 TURBO FLOW SWITCH"=FALSE, "HPD TURBO FLOW SWITCH"=FALSE, "Spare 7"=FALSE, "BTL ion gauge on signal"=FALSE, "BTL ion gauge degas signal"=FALSE, "TARGET ion gauge on signal"=FALSE, "TARGET ion gauge degas signal"=FALSE, "BTL2 ion gauge on signal"=FALSE, "BTL2 ion gauge degas signal"=FALSE, "HPD ion gauge on signal"=FALSE, "HPD ion gauge degas signal"=FALSE, "Spare 8"=FALSE, "Spare 9"=FALSE, "Spare 10"=FALSE, "Spare 11"=FALSE, "ROUGHING MANIFOLD VALVE"=FALSE, "BACKING MANIFOLD VALVE"=FALSE, "ROUGHING BACKING CONNECT VALVE"=FALSE, "BTL ROUGHING VALVE"=FALSE, "BTL VENT VALVE"=FALSE, "BTL Turbo Gate Valve"=FALSE, "BTL Turbo Backing Valve"=FALSE, "Roughing Manifold VV"=FALSE, "Backing Manifold VV"=FALSE, "TARGET ROUGHING VALVE"=FALSE, "BTL2 ROUGHING VALVE"=FALSE, "HPD ROUGHING VALVE"=FALSE, "GV BTL-TARGET"=FALSE, "GV TARGET-BTL2"=FALSE, "GV BTL2-HPD"=FALSE, "TARGET VENT VALVE"=FALSE, "BTL2 VENT VALVE"=FALSE, "HPD VENT VALVE"=FALSE, "TARGET  Turbo Gate Valve 1"=FALSE, "TARGET  Turbo Gate Valve 2"=FALSE, "BTL2 Turbo Gate Valve"=FALSE, "HPD  Turbo Gate Valve"=FALSE, "TARGET Turbo Backing Valve 1"=FALSE, "TARGET Turbo Backing Valve 2"=FALSE}, "EC statusboolarray3"={"BTL2 Turbo Backing Valve"=FALSE, "HPD Turbo Backing Valve"=FALSE, "Spare 1"=FALSE, "Spare 2"=FALSE, "Spare 3"=FALSE, "Spare 4"=FALSE, "Spare 5"=FALSE, "Spare 6"=FALSE, "Spare 7"=FALSE, "Spare 8"=FALSE, "Spare 9"=FALSE, "BTL Turbo Vent Valve"=FALSE, "TARGET1 Turbo Vent Valve"=FALSE, "TARGET2 Turbo Vent Valve"=FALSE, "BTL2 Turbo Vent Valve"=FALSE, "HPD Turbo Vent Valve"=FALSE, "Spare 10"=FALSE, "Spare 11"=FALSE, "BTL turbo pump run signal"=FALSE, "TARGET1 turbo pump run signal"=FALSE, "TARGET2 turbo pump run signal"=FALSE, "BTL2 turbo pump run signal"=FALSE, "HPD turbo pump run signal"=FALSE, "Spare 12"=FALSE, "watch dog timer - out"=FALSE, "BTL vented – out"=FALSE, "BTL medvac – out"=FALSE, "BTL hivac – out"=FALSE, "GPM EC - out"=FALSE, "GVM EC - out"=FALSE, "RP EC status - out"=FALSE, "RP LB toggle - out"=FALSE, "GATE ALL - closed out"=FALSE, "Spare 13"=FALSE, "Spare 14"=FALSE, "Spare 15"=FALSE, "Spare 16"=FALSE, "Spare 17"=FALSE, "Spare 18"=FALSE, "Spare 19"=FALSE, "Spare 20"=FALSE, "Spare 21"=FALSE, "Spare 22"=FALSE, "Spare 23"=FALSE, "Spare 24"=FALSE, "Spare 25"=FALSE, "Spare 26"=FALSE, "Spare 27"=FALSE}, "EC statusboolarray1"={"BTL ion gauge on feedback"=FALSE, "BTL ion gauge degas feedback"=FALSE, "TARGET ion gauge on feedback"=FALSE, "TARGET ion gauge degas feedback"=FALSE, "BTL2 ion gauge on feedback"=FALSE, "BTL2 ion gauge degas feedback"=FALSE, "HPD ion gauge on feedback"=FALSE, "HPD ion gauge degas feedback"=FALSE, "Spare 1"=FALSE, "Spare 2"=FALSE, "Spare 3"=FALSE, "Spare 4"=FALSE, "ROUGHING MANIFOLD VALVE opened"=FALSE, "ROUGHING MANIFOLD VALVE closed"=FALSE, "BACKING MANIFOLD VALVE opened"=FALSE, "BACKING MANIFOLD VALVE closed"=FALSE, "ROUGHING BACKING CONNECT VALVE opened"=FALSE, "ROUGHING BACKING CONNECT VALVE closed"=FALSE, "BTL ROUGHING VALVE opened"=FALSE, "BTL ROUGHING VALVE closed"=FALSE, "BTL VENT VALVE opened"=FALSE, "BTL VENT VALVE closed"=FALSE, "BTL Turbo Gate Valve opened"=FALSE, "BTL Turbo Gate Valve closed"=FALSE, "BTL Turbo Backing Valve opened"=FALSE, "BTL Turbo Backing Valve closed"=FALSE, "Roughing Manifold VV opened"=FALSE, "Roughing Manifold VV closed"=FALSE, "Backing Manifold VV opened"=FALSE, "Backing Manifold VV closed"=FALSE, "TARGET ROUGHING VALVE opened"=FALSE, "TARGET ROUGHING VALVE closed"=FALSE, "BTL2 ROUGHING VALVE opened"=FALSE, "BTL2 ROUGHING VALVE closed"=FALSE, "HPD ROUGHING VALVE opened"=FALSE, "HPD ROUGHING VALVE closed"=FALSE, "GV BTL-TARGET opened"=FALSE, "GV BTL-TARGET closed"=FALSE, "GV TARGET-BTL2 opened"=FALSE, "GV TARGET-BTL2 closed"=FALSE, "GV BTL2-HPD opened"=FALSE, "GV BTL2-HPD closed"=FALSE, "TARGET VENT VALVE opened"=FALSE, "TARGET VENT VALVE closed"=FALSE, "BTL2 VENT VALVE opened"=FALSE, "BTL2 VENT VALVE closed"=FALSE, "HPD VENT VALVE opened"=FALSE, "HPD VENT VALVE closed"=FALSE, "TARGET  Turbo Gate Valve 1 opened"=FALSE, "TARGET  Turbo Gate Valve 1 closed"=FALSE, "TARGET  Turbo Gate Valve 2 opened"=FALSE, "TARGET  Turbo Gate Valve 2 closed"=FALSE, "BTL2 Turbo Gate Valve opened"=FALSE, "BTL2 Turbo Gate Valve closed"=FALSE, "HPD  Turbo Gate Valve opened"=FALSE, "HPD  Turbo Gate Valve closed"=FALSE, "TARGET Turbo Backing Valve 1 opened"=FALSE, "TARGET Turbo Backing Valve 1 closed"=FALSE, "TARGET Turbo Backing Valve 2 opened"=FALSE, "TARGET Turbo Backing Valve 2 closed"=FALSE, "BTL2 Turbo Backing Valve opened"=FALSE, "BTL2 Turbo Backing Valve closed"=FALSE, "HPD Turbo Backing Valve opened"=FALSE, "HPD Turbo Backing Valve closed"=FALSE}, "EC statusintegerarray"={"BTL vacuum status word convectron ATM"=0, "TARGET vacuum status word convectron ATM 2"=0, "BTL2 vacuum status word convectron ATM 3"=0, "HPD vacuum status word convectron ATM 4"=0, "Spare 1"=0, "Spare 2"=0, "roughing pump vacuum status word convectron"=0, "backing pump vacuum status word convectron"=0, "roughing manifold vacuum status word convectron"=0, "backing manifold vacuum status word convectron"=0, "BTL Convectron vacuum status word convectron"=0, "TARGET1 Convectron vacuum status word convectron"=0, "TARGET2 Convectron vacuum status word convectron"=0, "BTL2 Convectron vacuum status word convectron"=0, "HPD Convectron vacuum status word convectron"=0, "BTL status word turbo pump"=0, "TARGET1 status word turbo pump"=0, "TARGET2 status word turbo pump"=0, "BTL2 status word turbo pump??"=0, "HPD status word turbo pump"=0, "Spare 3"=0, "Spare 4"=0, "Spare 5"=0, "Spare 6"=0, "BTL CONVECTRON Consolidate"=0, "Spare 7"=0, "Spare 8"=0, "Spare 9"=0, "TARGET Consolidate"=0, "Spare 10"=0, "Spare 11"=0, "Spare 12"=0, "BTL2 Consolidate"=0, "Spare 13"=0, "Spare 14"=0, "Spare 15"=0, "HPD Consolidate"=0, "Spare 16"=0, "Spare 17"=0, "Spare 18"=0, "Spare 19"=0, "Spare 20"=0, "Spare 21"=0, "Spare 22"=0, "Spare 23"=0, "Spare 24"=0, "Spare 25"=0, "Spare 26"=0}, "EC statusfloatarray"={"BTL READING ION GAUGE"=0.0, "TARGET READING ION GAUGE"=0.0, "BTL2 READING ION GAUGE"=0.0, "HPD READING ION GAUGE"=0.0, "Spare 1"=0.0, "Spare 2"=0.0, "Spare 3"=0.0, "Spare 4"=0.0, "roughing pump READING CONVECTRON GAUGE"=0.0, "backing pump READING CONVECTRON GAUGE"=0.0, "roughing manifold READING CONVECTRON GAUGE"=0.0, "backing manifold READING CONVECTRON GAUGE"=0.0, "BTL Convectron READING CONVECTRON GAUGE"=0.0, "TARGET1 READING CONVECTRON GAUGE"=0.0, "TARGET2 READING CONVECTRON GAUGE"=0.0, "BTL2 READING CONVECTRON GAUGE"=0.0, "HPD READING CONVECTRON GAUGE"=0.0, "Spare 5"=0.0, "Spare 6"=0.0, "Spare 7"=0.0, "Spare 8"=0.0, "Spare 9"=0.0, "Spare 10"=0.0, "Spare 11"=0.0}}  # EC Status Named
  w7 = T19 {"EC Command array 1"={"ROUGHING MANIFOLD VALVE"=FALSE, "BACKING MANIFOLD VALVE"=FALSE, "ROUGHING BACKING CONNECT VALVE"=FALSE, "BTL ROUGHING VALVE"=FALSE, "BTL VENT VALVE"=FALSE, "BTL Turbo Gate Valve"=FALSE, "BTL Turbo Backing Valve"=FALSE, "Roughing Manifold VV"=FALSE, "Backing Manifold VV"=FALSE, "TARGET ROUGHING VALVE"=FALSE, "BTL2 ROUGHING VALVE"=FALSE, "HPD ROUGHING VALVE"=FALSE, "GV BTL-TARGET"=FALSE, "GV TARGET-BTL2"=FALSE, "GV BTL2-HPD"=FALSE, "TARGET VENT VALVE"=FALSE}, " EC Command array 2"={"BTL2 VENT VALVE"=FALSE, "HPD VENT VALVE"=FALSE, "TARGET  Turbo Gate Valve 1"=FALSE, "TARGET  Turbo Gate Valve 2"=FALSE, "BTL2 Turbo Gate Valve"=FALSE, "HPD  Turbo Gate Valve"=FALSE, "TARGET Turbo Backing Valve 1"=FALSE, "TARGET Turbo Backing Valve 2"=FALSE, "BTL2 Turbo Backing Valve"=FALSE, "HPD Turbo Backing Valve"=FALSE, "Spare 1"=FALSE, "Spare 2"=FALSE, "ROUGHING PUMP"=FALSE, "BACKING PUMP"=FALSE, "Spare 3"=FALSE, "Spare 4"=FALSE}, "EC Command array 3"={"Spare 1"=FALSE, "Spare 2"=FALSE, "Spare 3"=FALSE, "BTL Turbo Vent Valve"=FALSE, "TARGET1 Turbo Vent Valve"=FALSE, "TARGET2 Turbo Vent Valve"=FALSE, "BTL2 Turbo Vent Valve"=FALSE, "HPD Turbo Vent Valve"=FALSE, "Spare 4"=FALSE, "Spare 5"=FALSE, "GPM"=FALSE, "GVM"=FALSE, "Spare 6"=FALSE, "BTL turbo pump"=FALSE, "TARGET1 turbo pump"=FALSE, "TARGET2 turbo pump"=FALSE}, "EC Command array 4"={"BLT turbo pump"=FALSE, "HPD turbo pump"=FALSE, "Spare 1"=FALSE, "BTL ION GAUGE ion gauge"=FALSE, "BTL ION GAUGE  ion gauge degas"=FALSE, "TARGET ion gauge"=FALSE, "TARGET ion gauge degas"=FALSE, "BTL2 ion gauge"=FALSE, "BTL2 ion gauge degas"=FALSE, "HPD ion gauge"=FALSE, "HPD ion gauge degas"=FALSE, "Spare 2"=FALSE, "Spare 3"=FALSE, "Spare 4"=FALSE, "Spare 5"=FALSE, "Spare 6"=FALSE}}  # EC Command Named
  w4 = T20 {"boolarray1"={FALSE, FALSE, FALSE, FALSE, FALSE, FALSE, FALSE, FALSE, FALSE, FALSE, FALSE, FALSE, FALSE, FALSE, FALSE, FALSE}, "boolarray2"={FALSE, FALSE, FALSE, FALSE, FALSE, FALSE, FALSE, FALSE, FALSE, FALSE, FALSE, FALSE, FALSE, FALSE, FALSE, FALSE}, "boolarray3"={FALSE, FALSE, FALSE, FALSE, FALSE, FALSE, FALSE, FALSE, FALSE, FALSE, FALSE, FALSE, FALSE, FALSE, FALSE, FALSE}, "boolarray4"={FALSE, FALSE, FALSE, FALSE, FALSE, FALSE, FALSE, FALSE, FALSE, FALSE, FALSE, FALSE, FALSE, FALSE, FALSE, FALSE}}  # LB Command Cluster
  w5 = T21 {"bits 2"=[FALSE, FALSE, FALSE, FALSE, FALSE, FALSE, FALSE, FALSE, FALSE, FALSE, FALSE, FALSE, FALSE, TRUE, FALSE, TRUE, FALSE, TRUE, FALSE, FALSE, FALSE, TRUE, FALSE, TRUE, FALSE, TRUE, FALSE, TRUE, FALSE, TRUE, TRUE, FALSE, TRUE, FALSE, FALSE, FALSE, FALSE, TRUE, FALSE, TRUE, FALSE, TRUE, FALSE, FALSE, FALSE, TRUE, FALSE, TRUE, FALSE, FALSE, FALSE, TRUE, FALSE, TRUE, FALSE, TRUE, FALSE, TRUE, FALSE, FALSE, FALSE, FALSE, FALSE, FALSE], "bits 2"=[FALSE, FALSE, FALSE, FALSE, FALSE, FALSE, FALSE, FALSE, FALSE, FALSE, TRUE, FALSE, TRUE, FALSE, FALSE, FALSE, FALSE, FALSE, FALSE, FALSE, TRUE, TRUE, FALSE, TRUE, TRUE, FALSE, FALSE, FALSE, FALSE, FALSE, FALSE, FALSE, FALSE, FALSE, FALSE, FALSE, FALSE, FALSE, FALSE, FALSE, FALSE, FALSE, FALSE, FALSE, FALSE, FALSE, FALSE, FALSE, FALSE, TRUE, TRUE, FALSE, FALSE, FALSE, FALSE, FALSE, FALSE, FALSE, FALSE, FALSE, FALSE, FALSE, FALSE, FALSE], "bits 2"=[FALSE, FALSE, FALSE, FALSE, FALSE, FALSE, FALSE, FALSE, FALSE, FALSE, FALSE, FALSE, FALSE, FALSE, FALSE, FALSE, FALSE, FALSE, FALSE, FALSE, FALSE, FALSE, FALSE, FALSE, TRUE, FALSE, TRUE, TRUE, FALSE, FALSE, FALSE, FALSE, FALSE, FALSE, FALSE, FALSE, FALSE, FALSE, FALSE, FALSE, FALSE, FALSE, FALSE, FALSE, FALSE, FALSE, FALSE, FALSE], [0, 0, 0, 0, 0, 0, 0, 0, 0, 0, 0, 0, 0, 0, 1, 3, 0, 0, 3, 3, 3, 3, 0, 0, 14126, 13880, 17707, 12338, 14126, 14642, 17707, 12338, 14126, 14135, 17707, 12338, 14382, 12600, 17707, 12338, 0, 0, 0, 0, 0, 0, 0, 0], "FLOAT NUMBERS 2"=[1.7352603e-06, 0.9935997, 0.9935997, 0.19649225, 0.0051960573, 0.00032194593, 0.0, 0.0, 693.9616, 709.14777, 703.4565, 718.4583, 67.805214, 604.4024, 628.84827, 47.743088, 0.28528655, 42.802475, 27.788507, 50.719826, 0.0, 0.0, 0.0, 0.0]}  # LB Status
  w8 = T20 {"boolarray1"={FALSE, FALSE, FALSE, FALSE, FALSE, FALSE, FALSE, FALSE, FALSE, FALSE, FALSE, FALSE, FALSE, FALSE, FALSE, FALSE}, "boolarray2"={FALSE, FALSE, FALSE, FALSE, FALSE, FALSE, FALSE, FALSE, FALSE, FALSE, FALSE, FALSE, FALSE, FALSE, FALSE, FALSE}, "boolarray3"={FALSE, FALSE, FALSE, FALSE, FALSE, FALSE, FALSE, FALSE, FALSE, FALSE, FALSE, FALSE, FALSE, FALSE, FALSE, FALSE}, "boolarray4"={FALSE, FALSE, FALSE, FALSE, FALSE, FALSE, FALSE, FALSE, FALSE, FALSE, FALSE, FALSE, FALSE, FALSE, FALSE, FALSE}}  # EC Command Cluster
  w10 = T22 {"Source_URL EC"="192.168.13.66", "Target_URL EC"="192.168.13.66", "Source_URL LB"="192.168.13.98", "Target_URL LB"="192.168.13.98"}  # Connection URLs
  w11 = T23 {"Status TCP Connection EC"=refnum, "Command TCP Connection EC"=refnum, "Status TCP Connection LB"=refnum, "Command TCP Connection LB"=refnum}  # TCPConnection
  w12 = T21 {"bits 2"=[FALSE, FALSE, FALSE, FALSE, FALSE, FALSE, FALSE, FALSE, FALSE, FALSE, FALSE, FALSE, FALSE, TRUE, FALSE, TRUE, FALSE, TRUE, FALSE, FALSE, FALSE, TRUE, FALSE, TRUE, FALSE, TRUE, FALSE, TRUE, FALSE, TRUE, TRUE, FALSE, TRUE, FALSE, FALSE, FALSE, FALSE, TRUE, FALSE, TRUE, FALSE, TRUE, FALSE, FALSE, FALSE, TRUE, FALSE, TRUE, FALSE, FALSE, FALSE, TRUE, FALSE, TRUE, FALSE, TRUE, FALSE, TRUE, FALSE, FALSE, FALSE, FALSE, FALSE, FALSE], "bits 2"=[FALSE, FALSE, FALSE, FALSE, FALSE, FALSE, FALSE, FALSE, FALSE, FALSE, TRUE, FALSE, TRUE, FALSE, FALSE, FALSE, FALSE, FALSE, FALSE, FALSE, TRUE, TRUE, FALSE, TRUE, TRUE, FALSE, FALSE, FALSE, FALSE, FALSE, FALSE, FALSE, FALSE, FALSE, FALSE, FALSE, FALSE, FALSE, FALSE, FALSE, FALSE, FALSE, FALSE, FALSE, FALSE, FALSE, FALSE, FALSE, FALSE, TRUE, TRUE, FALSE, FALSE, FALSE, FALSE, FALSE, FALSE, FALSE, FALSE, FALSE, FALSE, FALSE, FALSE, FALSE], "bits 2"=[FALSE, FALSE, FALSE, FALSE, FALSE, FALSE, FALSE, FALSE, FALSE, FALSE, FALSE, FALSE, FALSE, FALSE, FALSE, FALSE, FALSE, FALSE, FALSE, FALSE, FALSE, FALSE, FALSE, FALSE, TRUE, FALSE, TRUE, TRUE, FALSE, FALSE, FALSE, FALSE, FALSE, FALSE, FALSE, FALSE, FALSE, FALSE, FALSE, FALSE, FALSE, FALSE, FALSE, FALSE, FALSE, FALSE, FALSE, FALSE], [0, 0, 0, 0, 0, 0, 0, 0, 0, 0, 0, 0, 0, 0, 1, 3, 0, 0, 3, 3, 3, 3, 0, 0, 14126, 13880, 17707, 12338, 14126, 14642, 17707, 12338, 14126, 14135, 17707, 12338, 14382, 12600, 17707, 12338, 0, 0, 0, 0, 0, 0, 0, 0], "FLOAT NUMBERS 2"=[1.7352603e-06, 0.9935997, 0.9935997, 0.19649225, 0.0051960573, 0.00032194593, 0.0, 0.0, 693.9616, 709.14777, 703.4565, 718.4583, 67.805214, 604.4024, 628.84827, 47.743088, 0.28528655, 42.802475, 27.788507, 50.719826, 0.0, 0.0, 0.0, 0.0]}  # EC Status
  w13 = T24 {"Current VI Reference"=refnum, "Close Panel on Exit?"=FALSE}  # Core
  n1 = Bundle("Isolate HPBD"=w1, "Core"=w13, "Status Display Array"=w2, "Connection URLs"=w10, "EC Status"=w12, "EC Status Named"=w9, "TCPConnection"=w11, "EC Command Cluster"=w8, "EC Command Named"=w7, "LB Status Named"="LB Status Named", "LB Status"=w5, "LB Command Cluster"=w4, "LB Command Named"=w3) -> ()  [unwired: 1 in, 1 out]
